vi "get_cluster_from_config.vi"(4 "error in (no error)":errorcluster, 6 "microscope tag type":string, 7 "path to config file":path) -> (0 "error out":errorcluster, 3 "Array":T1(array[cluster]))   [LabVIEW 2010, in "XML_repo_library.lvlib"]
uses:
  XML_repo_library.lvlib
  <vilib>/xml/Load XML File.vi
  <vilib>/xml/Close Reference(Node).vi
  <vilib>/xml/NI_XML.lvlib
  C:/Program Files (x86)/National Instruments/LabVIEW 2010/resource/objmgr/DOMUserDefRef.rc
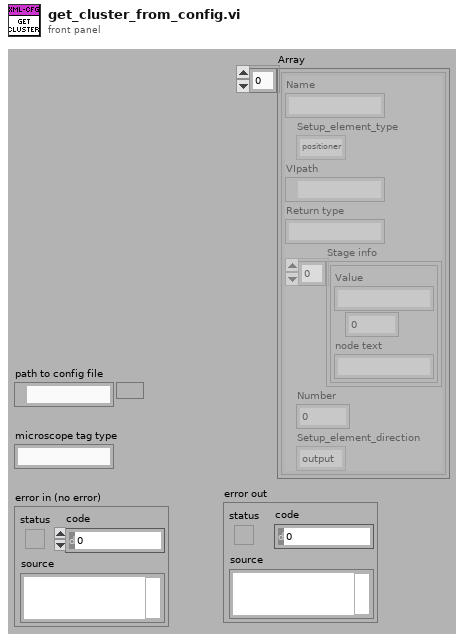
[diagram p1: front panel]
types:
  T1 = cluster{"Name":string, "Setup_element_type":enum16{"positioner", "acquisition", "synchronized"}, "VIpath":path, "Return type":string, "Stage info":cluster{"Value":string, i32, "node text":string}[], "Number":u32, "Setup_element_direction":enum16{"output", "input", "io"}}[]
  T2 = cluster{"Name":string, "Setup_element_type":enum16{"positioner", "acquisition", "synchronized"}, "VIpath":path, "Return type":string, "Stage info":cluster{"Value":string, i32, "node text":string}[], "Number":u32, "Setup_element_direction":enum16{"output", "input", "io"}}
  T3 = enum16{"positioner", "acquisition", "synchronized"}
  T4 = cluster{"Value":string, i32, "node text":string}[]
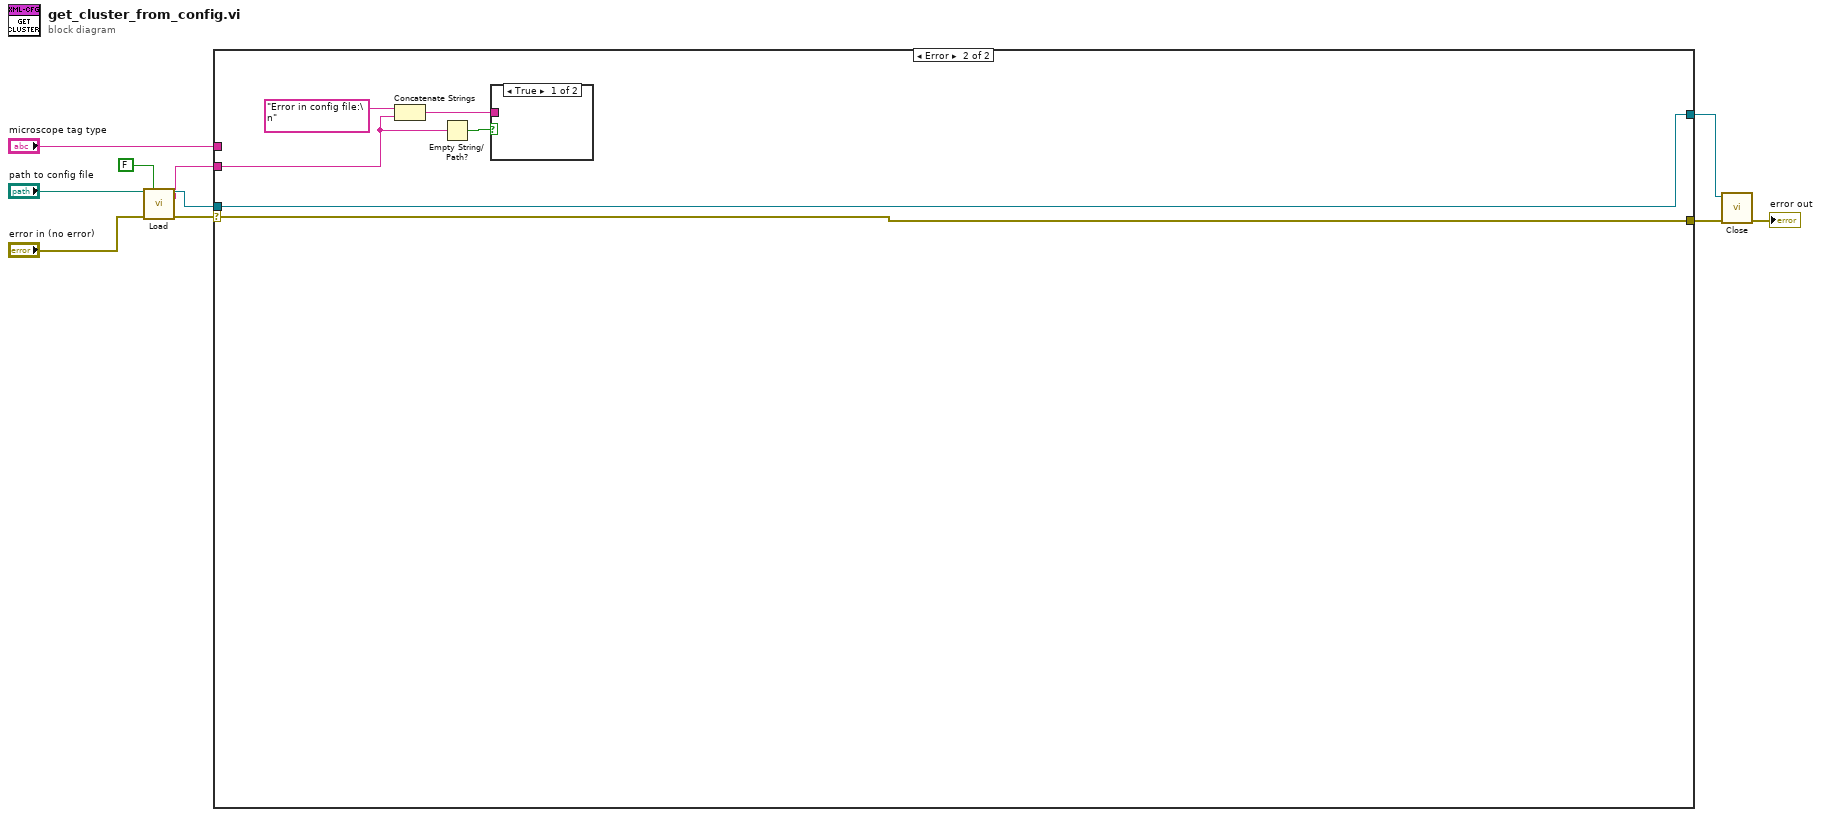
[diagram p0: block diagram]
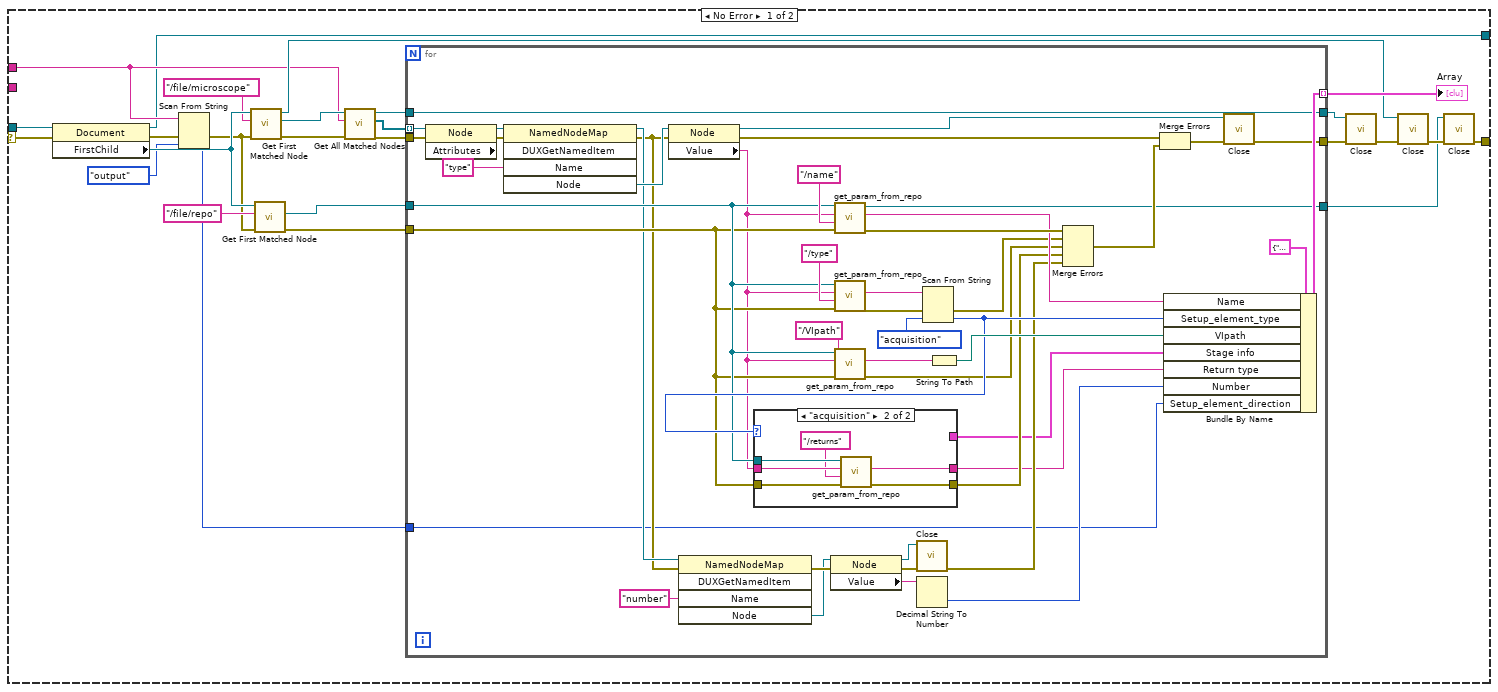
[diagram p2: hidden frame]
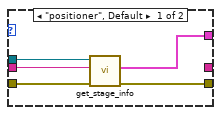
[diagram p3: hidden frame]
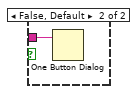
[diagram p4: hidden frame]
diagram:
  n1 = call-poly <vilib>:"Load.vi"("path to XML document"="path to config file", "preserve whitespace (True)"=FALSE, "error in (no error)"="error in (no error)") -> ("DOM document out"=w8:refnum<k20>, "parse errors"=w2:string, "error out"=w1:errorcluster)  [unwired: 10 in]
  n2 = case shown="Error" w1 {
    selector: w1 -> [w11 w96]
    tunnel: w8 -> [w25 w98]
    tunnel: [w19 w96] -> w6
    tunnel: "microscope tag type" -> [w17 _]
    tunnel: [w13 w98] -> w3
    tunnel: w2 -> [_ w93]
    frame No Error {
      n3 = property class="Document"(reference=w25, error in=w11) -> (reference out=w13:refnum<k20>, error out=w16:errorcluster, "FirstChild"=w24:refnum<k20>)
      n4 = Scan From String(input string=w17, error in=w16, default 1=enum16{"output", "input", "io"}."output" ("Enum")) -> (error out=w15:errorcluster, output 1=w14:enum16{"output", "input", "io"})  [unwired: 2 in, 2 out]
      n5 = call <vilib>:"Get First Matched Node.vi"("error in (no error)"=w15, "XPath expression"="/file/microscope", "node in"=w24) -> ("error out"=w28:errorcluster, "node result"=w27:refnum<k20>, "node out"=w34:refnum<k20>)  [unwired: 6 in]
      n6 = call <vilib>:"Get First Matched Node.vi"("error in (no error)"=w15, "XPath expression"="/file/repo", "node in"=w24) -> ("error out"=w23:errorcluster, "node result"=w22:refnum<k20>)  [unwired: 6 in, 1 out]
      n7 = call <vilib>:"Get All Matched Nodes.vi"("error in (no error)"=w28, "XPath expression"=w17, "node in"=w27) -> ("error out"=w26:errorcluster, "node result array"=w29:refnum<k20>[], "node out"=w30:refnum<k20>)  [unwired: 6 in]
      n8 = for {
        tunnel: w29 -> [w81] mode=indexing
        tunnel: w26 -> [w80]
        tunnel: w22 -> [w64]
        tunnel: w23 -> [w63]
        tunnel: [w47] -> w31
        tunnel: [w72] -> w36 mode=indexing
        tunnel: [w71] -> w32
        tunnel: w30 -> [w71]
        tunnel: [w54] -> w12
        tunnel: w14 -> [w38]
        n9 = property class="Node"(reference=w81, error in=w80) -> (error out=w79:errorcluster, "Attributes"=w78:refnum<k20>)  [unwired: 1 out]
        n10 = invoke class="NamedNodeMap" method="DUXGetNamedItem"(reference=w78, error in=w79, "Name"="type") -> (reference out=w53:refnum<k20>, error out=w52:errorcluster, "Node"=w76:refnum<k20>)  [unwired: 2 in, 2 out]
        n11 = property class="Node"(reference=w76, error in=w52) -> (reference out=w46:refnum<k20>, error out=w75:errorcluster, "Value"=w62:string)
        n12 = invoke class="NamedNodeMap" method="DUXGetNamedItem"(reference=w53, error in=w52, "Name"="number") -> (error out=w50:errorcluster, "Node"=w49:refnum<k20>)  [unwired: 2 in, 3 out]
        n13 = property class="Node"(reference=w49, error in=w50) -> (reference out=w45:refnum<k20>, error out=w43:errorcluster, "Value"=w44:string)
        n14 = call "get_param_from_repo.vi"("error in (no error)"=w63, "param_name"="/name" ("string"), "repo_type"=w62, "node in"=w64) -> ("error out"=w68:errorcluster, "parameter"=w67:string, "node out"=w54:refnum<k20>)  [unwired: 5 in]
        n15 = call "get_param_from_repo.vi"("error in (no error)"=w63, "param_name"="/type" ("string"), "repo_type"=w62, "node in"=w64) -> ("error out"=w57:errorcluster, "parameter"=w65:string)  [unwired: 5 in, 1 out]
        n16 = call "get_param_from_repo.vi"("error in (no error)"=w63, "param_name"="/VIpath" ("string"), "repo_type"=w62, "node in"=w64) -> ("error out"=w60:errorcluster, "parameter"=w59:string)  [unwired: 5 in, 1 out]
        n17 = call-poly <vilib>:"Close.vi"("error in (no error)"=w43, "node"=w45) -> ("error out"=w42:errorcluster)  [unwired: 7 in]
        n18 = Decimal String To Number(string=w44) -> (number=w41:i32)  [unwired: 2 in, 1 out]
        n19 = Scan From String(input string=w65, error in=w57, default 1=T3."acquisition" ("Setup_element")) -> (error out=w56:errorcluster, output 1=w70:T3)  [unwired: 2 in, 2 out]
        n20 = case shown="\"acquisition\"" w70 {
          tunnel: w64 -> [w83 w92]
          tunnel: w63 -> [w86 w89]
          tunnel: w62 -> [w84 w91]
          tunnel: [_ w88] -> w39
          tunnel: [w85 w87] -> w58
          tunnel: [w82 _] -> w40
          frame "positioner", Default {
            n21 = call "get_stage_info.vi"("error in (no error)"=w86, "repo_type"=w84, "node in"=w83) -> ("error out"=w85:errorcluster, "Stage info"=w82:T4)  [unwired: 6 in, 1 out]
          }
          frame "acquisition" {
            n22 = call "get_param_from_repo.vi"("error in (no error)"=w89, "param_name"="/returns" ("string"), "repo_type"=w91, "node in"=w92) -> ("error out"=w87:errorcluster, "parameter"=w88:string)  [unwired: 5 in, 1 out]
          }
        }
        n23 = String To Path(string=w59) -> (path=w73:path)
        n24 = Merge Errors(w68, w56, w60, w58, w42) -> (w55:errorcluster)
        n25 = Merge Errors(w75, w55) -> (w48:errorcluster)
        n26 = Bundle By Name(cluster=T2 {"Name"="", "Setup_element_type"=enum."positioner", "VIpath"=path "", "Return type"="", "Stage info"=[], "Number"=0, "Setup_element_direction"=enum."output"} ("Setup_element_cluster"), "Name"=w67, "Setup_element_type"=w70, "VIpath"=w73, "Stage info"=w40, "Return type"=w39, "Number"=w41, "Setup_element_direction"=w38) -> (w72:T2)
        n27 = call-poly <vilib>:"Close.vi"("error in (no error)"=w48, "node"=w46) -> ("error out"=w47:errorcluster)  [unwired: 7 in]
      }
      "Array" <- w36
      n28 = call-poly <vilib>:"Close.vi"("error in (no error)"=w31, "node"=w32) -> ("error out"=w33:errorcluster)  [unwired: 7 in]
      n29 = call-poly <vilib>:"Close.vi"("error in (no error)"=w33, "node"=w34) -> ("error out"=w35:errorcluster)  [unwired: 7 in]
      n30 = call-poly <vilib>:"Close.vi"("error in (no error)"=w35, "node"=w12) -> ("error out"=w19:errorcluster)  [unwired: 7 in]
    }
    frame Error {
      n31 = Concatenate Strings("Error in config file:\n" ("string"), w93) -> (w95:string)
      n32 = Empty String/Path?(string/path=w93) -> (empty?=w94:bool)
      n33 = case shown="True" w94 {
        tunnel: w95 -> [_ w99]
        frame True {
        }
        frame False, Default {
          n34 = One Button Dialog(message=w99) -> ()  [unwired: 1 in, 1 out]
        }
      }
    }
  }
  n35 = call-poly <vilib>:"Close.vi"("error in (no error)"=w6, "node"=w3) -> ("error out"=→"error out":errorcluster)  [unwired: 7 in]
